vi "Auto-adjust rectangle size.vi"(9 "Center around clicked pixel (F)":bool, 11 "New Coordinates":i32[](array[numeric])) -> (3 "Modified coordinates":i32[](array[numeric]))   [LabVIEW 2017]
uses:
  Globals/gl_ROI Entry UI globals.vi
panel:
  out "Last length on Y":i32
  out "Last length on X":i32
  # "X1\nY1\nX2\nY2"
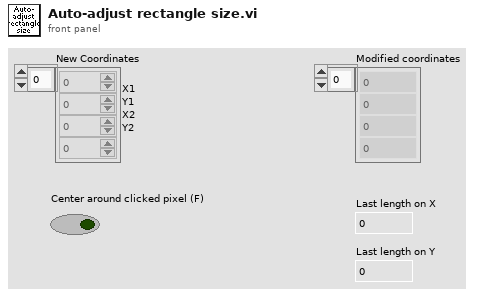
[diagram p1: front panel]
types:
  T1 = typedef "ROI entry screen ctrl refs cluster.ctl" = cluster{"Done button":refnum<vi>, "Imaging button":refnum<vi>, "Acquisition button":refnum<vi>, "POI dwell time (us)":refnum<vi>, "Scan dwell time per pixel (us)":refnum<vi>, "# of planes":refnum<vi>, "Zoom Ctrl":refnum<vi>, "Equal size":refnum<vi>, "Channel":refnum<vi>, "Image Display":refnum<vi>, "Z-Plane Selector":refnum<vi>, "Number of lines left":refnum<vi>, "Z-stack folder path":refnum<vi>, "POI Density":refnum<vi>, "Arb Plane Entry":refnum<vi>, "Whole plane":refnum<vi>, "Clear Last":refnum<vi>, "Clear All":refnum<vi>, "Trial Length (sec)":refnum<vi>, "Palette Type":refnum<vi>, "Intensity slider":refnum<vi>, "# POI":refnum<vi>, "Max Z Proj":refnum<vi>, "Zplane ind":refnum<vi>, "Wavelength (nm)":refnum<vi>, "Number of Trials":refnum<vi>, "Funct stim.trig.enable":refnum<vi>, "Funct stim.trig.delay (s)":refnum<vi>, "Line Mode":refnum<vi>, "Step size (µm)":refnum<vi>, "ROI move mode":refnum<vi>, "Cool-down time (s)":refnum<vi>, "Enable cool-down time":refnum<vi>, "Motor Z ind. (um)":refnum<vi>, "AOL Z ind. (um)":refnum<vi>, "Load Reference Image":refnum<vi>}
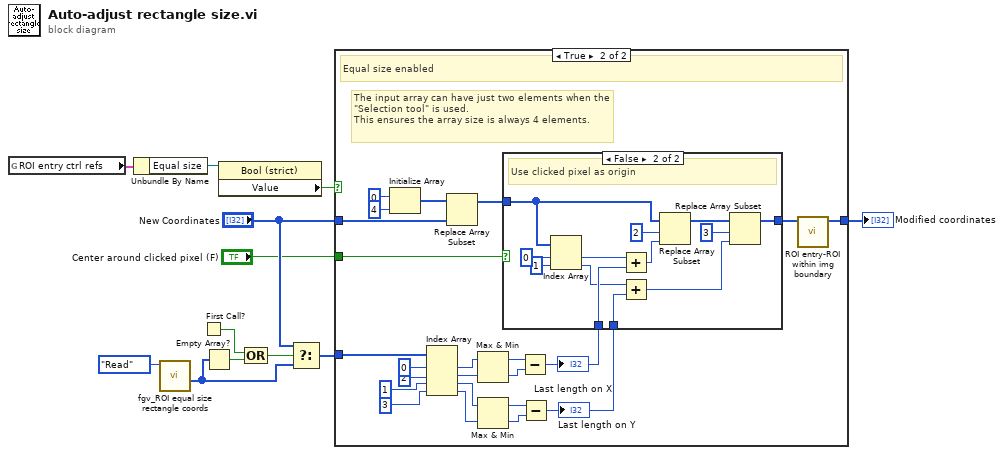
[diagram p0: block diagram]
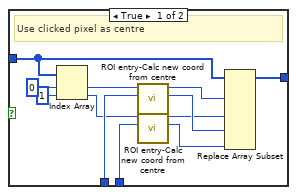
[diagram p3: hidden frame]
diagram:
  n1 = global read "gl_ROI Entry UI globals.vi" "ROI entry ctrl refs"() -> (w9:T1)
  n2 = Unbundle By Name(w9) -> ("Equal size"=w10:refnum<vi>)
  n3 = call "fgv_ROI equal size rectangle coords.vi"("Function"=enum16{"Intialize", "Write", "Read", "Clear"}."Read") -> ("Registered Rectangle Coordinates"=w5:i32[])  [unwired: 9 in, 1 out]
  n4 = First Call?() -> (First Call?: T/F=w3:bool)
  n5 = Empty Array?(array=w5) -> (empty?=w4:bool)
  n6 = property class="Bool (strict)"(reference=w10) -> ("Value"=w8:bool)  [unwired: 1 in, 2 out]
  n7 = Compound Arithmetic op=OR(w3, w4) -> (w2:bool)
  n8 = Select(t="New Coordinates", s=w2, f=w5) -> (s? t:f=w12:i32[])
  n9 = case shown="True" w8 {
    tunnel: "New Coordinates" -> [w13 w15]
    tunnel: w12 -> [_ w24]
    tunnel: [w13 w20] -> w7
    tunnel: "Center around clicked pixel (F)" -> [_ w14]
    frame False {
      # "Equal size disabled"
    }
    frame True {
      # "The input array can have just two elements when the \"Selection tool\" is used.\nThis ensures the array size is always 4 elements."
      # "Equal size enabled"
      n10 = Initialize Array(0 ("dimension size"), 4 ("dimension size")) -> (w17:i32[])
      n11 = Index Array(array=w24, index #1=0 ("index"), index #2=2 ("index"), index #3=1 ("index"), index #4=3 ("index")) -> (element #1=w22:i32, element #2=w34:i32, element #3=w28:i32, element #4=w27:i32)
      n12 = Replace Array Subset(array=w17, new element=w15) -> (w16:i32[])  [unwired: 1 in]
      n13 = Max & Min(x=w22, y=w34) -> (max(x,y)=w23:i32, min(x,y)=w33:i32)
      n14 = Max & Min(x=w28, y=w27) -> (max(x,y)=w29:i32, min(x,y)=w30:i32)
      n15 = Subtract(x=w23, y=w33) -> (x-y=w26:i32)
      "Last length on X" <- w26
      n16 = Subtract(x=w29, y=w30) -> (x-y=w25:i32)
      "Last length on Y" <- w25
      n17 = case shown="False" w14 {
        tunnel: w26 -> [w43 w53]
        tunnel: w25 -> [w39 w52]
        tunnel: [w46 w50] -> w21
        tunnel: w16 -> [w45 w49]
        frame True {
          # "Use clicked pixel as centre"
          n18 = Index Array(array=w45, index #1=0 ("index"), index #2=1 ("index")) -> (element #1=w44:i32, element #2=w40:i32)
          n19 = call "ROI entry-Calc new coord from centre.vi"("Previous length"=w43, "Central point coordinate"=w44) -> ("New max"=w41:i32, "New min"=w42:i32)  [unwired: 8 in]
          n20 = call "ROI entry-Calc new coord from centre.vi"("Previous length"=w39, "Central point coordinate"=w40) -> ("New max"=w37:i32, "New min"=w38:i32)  [unwired: 8 in]
          n21 = Replace Array Subset(array=w45, new element #1=w42, new element #2=w38, new element #3=w41, new element #4=w37) -> (w46:i32[])  [unwired: 4 in]
        }
        frame False {
          # "Use clicked pixel as origin"
          n22 = Index Array(array=w49, index #1=0 ("index"), index #2=1 ("index")) -> (element #1=w60:i32, element #2=w51:i32)
          n23 = Add(x=w60, y=w53) -> (x+y=w59:i32)
          n24 = Add(x=w51, y=w52) -> (x+y=w55:i32)
          n25 = Replace Array Subset(array=w49, new element=w59, index=2) -> (w54:i32[])
          n26 = Replace Array Subset(array=w54, new element=w55, index=3) -> (w50:i32[])
        }
      }
      n27 = call "ROI entry-ROI within img boundary.vi"("Coordinates in"=w21) -> ("Coordinates out"=w20:i32[])  [unwired: 10 in]
    }
  }
  "Modified coordinates" <- w7
